vi "Write to Port.vi"(10 "value":i16, 11 "AO in":refnum<class "AO1.lvclass">) -> ()   [LabVIEW 2017, in "Analog IO.lvlib" / "AO1.lvclass"]
uses:
  AO1.lvclass
  <vilib>/rvi/eio/common/nirviEmuTemplateMethod_errors.vi
  <vilib>/eio/EIONode/EIONode.xnode
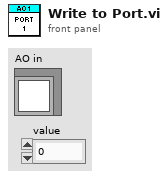
[diagram p1: front panel]
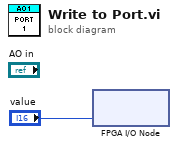
[diagram p0: block diagram]
diagram:
  n1 = xnode "FPGA I/O Node"("AO1"="value") -> ()  [unwired: 1 in, 1 out]
